vi "определение состояние пкомпрессоров.vi"(8 "забор":bool, 11 "Сжатие":bool) -> (3 "положение":string)   [LabVIEW 2011]
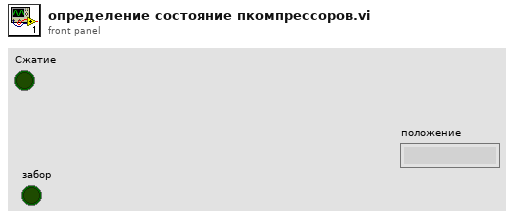
[diagram p1: front panel]
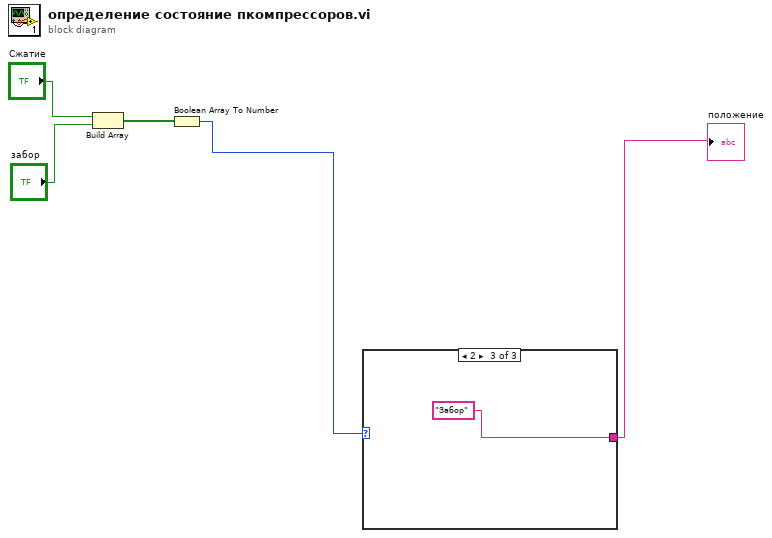
[diagram p0: block diagram]
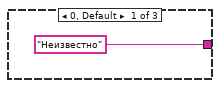
[diagram p2: hidden frame]
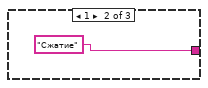
[diagram p3: hidden frame]
diagram:
  n1 = Build Array("Сжатие", "забор") -> (w3:bool[])
  n2 = Boolean Array To Number(Boolean array=w3) -> (number=w2:u32)
  n3 = case shown="2" w2 {
    tunnel: ["Неизвестно" "Сжатие" "Забор"] -> w1
    frame 0, Default {
    }
    frame 1 {
    }
    frame 2 {
    }
  }
  "положение" <- w1
